vi "Load.vi"(8 "error in (no error)":errorcluster, 10 "Data_IN":variant, 11 "_ConfigClass_INI_IN":refnum<class "_ConfigClass_INI.lvclass">) -> (0 "error out":errorcluster, 3 "_ConfigClass_INI_OUT":refnum<class "_ConfigClass_INI.lvclass">)   [LabVIEW 2019, in "_ConfigClass_INI.lvlib" / "_ConfigClass_INI.lvclass"]
uses:
  _ConfigClass_INI.lvclass
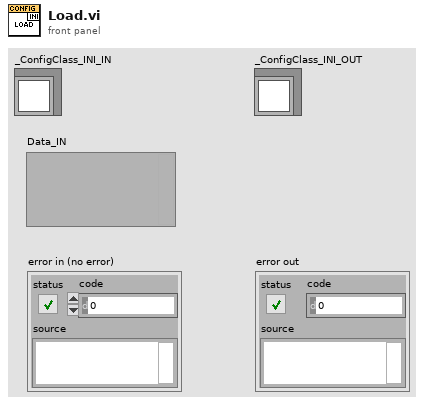
[diagram p1: front panel]
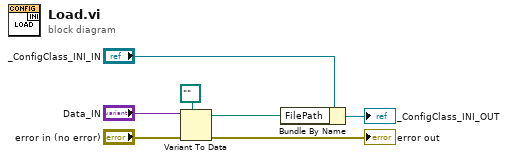
[diagram p0: block diagram]
diagram:
  n1 = Variant To Data(error in="error in (no error)", type=path "", Variant="Data_IN") -> (data=w3:path, error out=→"error out":errorcluster)
  n2 = Bundle By Name(cluster="_ConfigClass_INI_IN", "FilePath"=w3) -> (→"_ConfigClass_INI_OUT":refnum<class "_ConfigClass_INI.lvclass">)
